vi "construct_row.vi"(10 "input":T1, 11 "Array with C_raw, C_target":dbl[](array[numeric])) -> (3 "output":T1)   [LabVIEW 2019]
uses:
  RowData_Type.ctl
  enum_observed_clarified.ctl
panel:
  in  "DOM?":bool
  # "control if model should use DOM here"
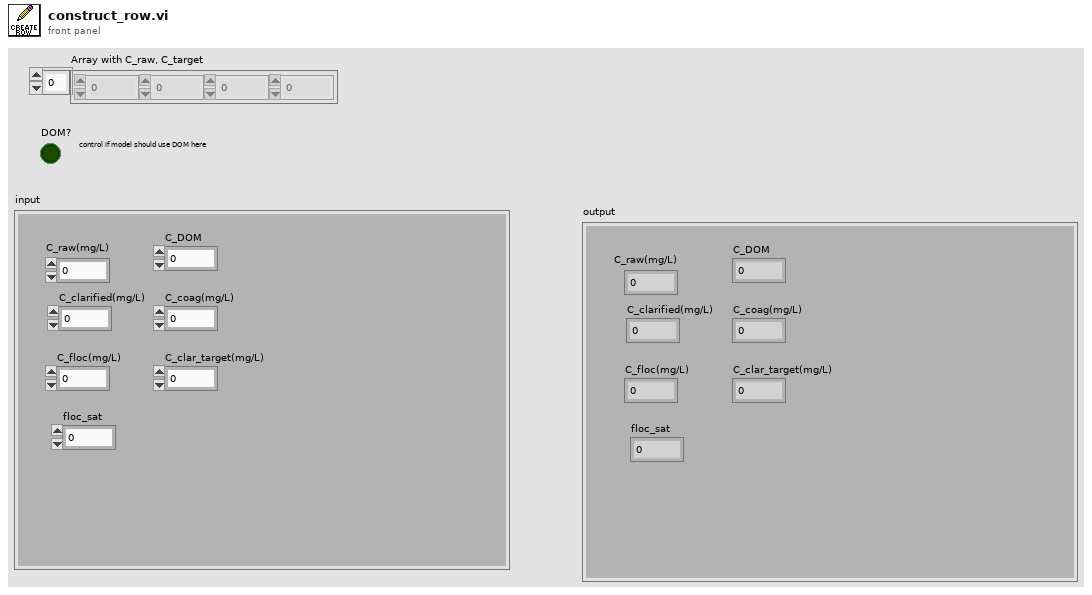
[diagram p1: front panel]
types:
  T1 = typedef "RowData_Type.ctl" = cluster{"C_raw(mg/L)":dbl, "C_clarified(mg/L)":dbl, "C_floc(mg/L)":dbl, "floc_sat":dbl, "C_DOM":dbl, "C_coag(mg/L)":dbl, "C_clar_target(mg/L)":dbl}
  T2 = typedef "enum_observed_clarified.ctl" = enum16{"Observed", "Target"}
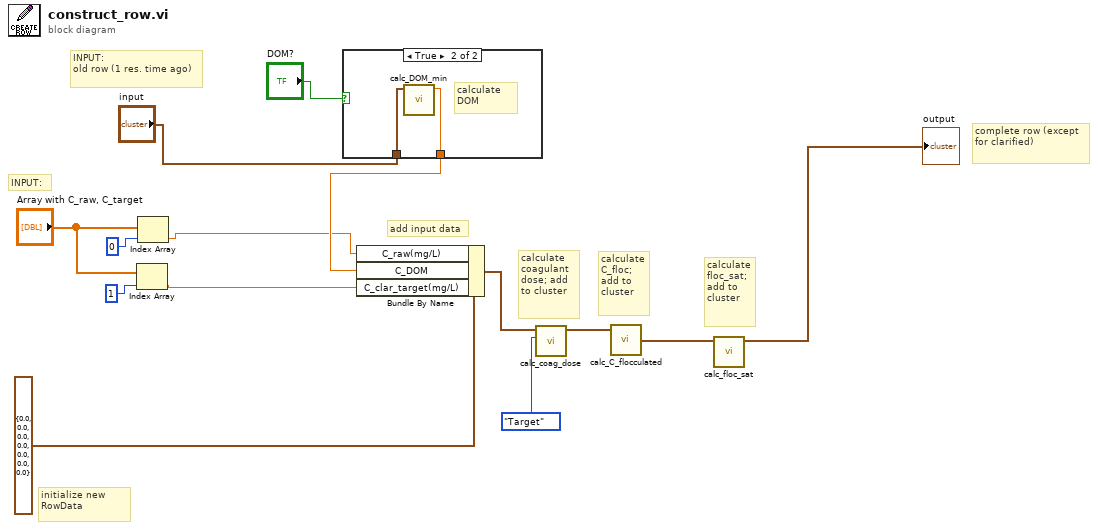
[diagram p0: block diagram]
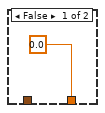
[diagram p2: hidden frame]
diagram:
  # "complete row (except for clarified)"
  # "INPUT:"
  # "INPUT:\nold row (1 res. time ago)"
  # "calculate floc_sat;\nadd to cluster"
  # "calculate\nC_floc; add to cluster"
  # "calculate coagulant dose; add to cluster"
  # "initialize new RowData"
  # "add input data"
  n1 = Index Array(array="Array with C_raw, C_target", index=1) -> (element=w1:dbl)
  n2 = Index Array(array="Array with C_raw, C_target", index=0) -> (element=w2:dbl)
  n3 = case shown="True" "DOM?" {
    tunnel: "input" -> [_ w17]
    tunnel: [0.0 w16] -> w6
    frame False {
    }
    frame True {
      # "calculate DOM"
      n4 = call "calc_DOM_min.vi"("Input RowData"=w17) -> ("DOM"=w16:dbl)  [unwired: 10 in]
    }
  }
  n5 = Bundle By Name(cluster=T1 {"C_raw(mg/L)"=0.0, "C_clarified(mg/L)"=0.0, "C_floc(mg/L)"=0.0, "floc_sat"=0.0, "C_DOM"=0.0, "C_coag(mg/L)"=0.0, "C_clar_target(mg/L)"=0.0} ("typedef_test"), "C_raw(mg/L)"=w2, "C_DOM"=w6, "C_clar_target(mg/L)"=w1) -> (w13:T1)
  n6 = call "calc_coag_dose.vi"("Enum"=enum_observed_clarified."Target", "RowData input"=w13) -> ("RowData output"=w11:T1)  [unwired: 9 in]
  n7 = call "calc_C_flocculated.vi"("RowData"=w11) -> ("RowData 2"=w10:T1)  [unwired: 2 in]
  n8 = call "calc_floc_sat.vi"("RowData"=w10) -> ("RowData 2"=→"output":T1)  [unwired: 10 in]
